vi "실습 2-1.vi"() -> ()   [LabVIEW 2014]
panel:
  out "데이터":timestamp
  in  "정지":bool
  in  "큐입력":bool
  out "설명":string
  out "큐 데이터":cluster{"설명":string, "데이터":variant}
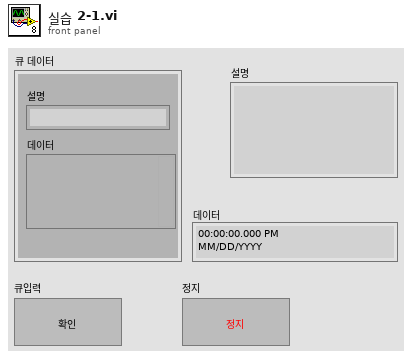
[diagram p1: front panel]
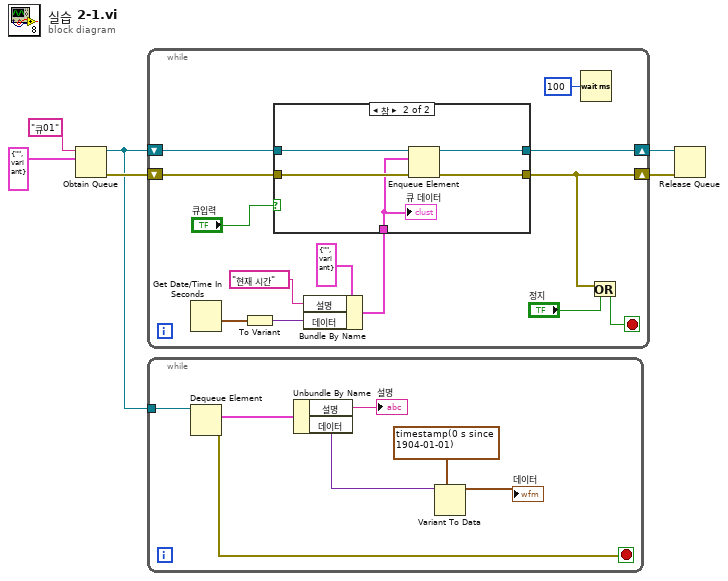
[diagram p0: block diagram]
diagram:
  n1 = Obtain Queue(name (unnamed)="큐01" ("이름(이름없음)"), element data type=cluster{"설명":string, "데이터":variant} {"설명"="", "데이터"=variant} ("큐 데이터")) -> (queue out=w1:refnum<queue>, error out=w4:errorcluster)  [unwired: 3 in, 1 out]
  n2 = while {
    shift-right: [w18] -> w2
    shift-left: w1 -> [w19]
    shift-right: [w13] -> w3
    shift-left: w4 -> [w17]
    stop <- w14 stop-if-true
    n3 = Get Date/Time In Seconds() -> (seconds since 1Jan1904=w9:timestamp)
    n4 = To Variant(anything=w9) -> (Variant=w7:variant)
    n5 = Bundle By Name(cluster=cluster{"설명":string, "데이터":variant} {"설명"="", "데이터"=variant} ("큐 데이터"), "설명"="현재 시간", "데이터"=w7) -> (w8:cluster{"설명":string, "데이터":variant})
    n6 = case shown="참" "큐입력" {
      tunnel: w19 -> [w21 w26]
      tunnel: [w21 w25] -> w18
      tunnel: w17 -> [w20 w24]
      tunnel: [w20 w23] -> w13
      tunnel: w8 -> [_ w22]
      frame False {
      }
      frame True {
        n7 = Enqueue Element(queue=w26, element=w22, error in (no error)=w24) -> (queue out=w25:refnum<queue>, error out=w23:errorcluster)  [unwired: 1 in, 1 out]
        "큐 데이터" <- w22
      }
    }
    n8 = Wait (ms)(milliseconds to wait=u32 100 ("대기 시간(ms)")) -> ()  [unwired: 1 out]
    n9 = Or(x=w13, y="정지") -> (x .or. y?=w14:bool)
  }
  n10 = while {
    tunnel: w1 -> [w33]
    stop <- w27 stop-if-true
    n11 = Dequeue Element(queue=w33) -> (element=w32:cluster{"설명":string, "데이터":variant}, error out=w27:errorcluster)  [unwired: 2 in, 2 out]
    n12 = Unbundle By Name(w32) -> ("설명"=→"설명":string, "데이터"=w30:variant)
    n13 = Variant To Data(type=timestamp(0 s since 1904-01-01), Variant=w30) -> (data=→"데이터":timestamp)  [unwired: 1 in, 1 out]
  }
  n14 = Release Queue(queue=w2, error in (no error)=w3) -> ()  [unwired: 1 in, 3 out]
